vi "CVTTraceUpdate.vi"(8 "error in (no error)":errorcluster, 10 "Channels":string[](array[string]), 11 "TektronixDPOSimple in":refnum<class "Tektronix MDO MSO DPO.lvclass">) -> (0 "error out":errorcluster, 2 "CommandOut":string, 3 "TektronixDPOSimple out":refnum<class "Tektronix MDO MSO DPO.lvclass">)   [LabVIEW 2020, in "Tektronix MDO MSO DPO.lvclass"]
uses:
  Tektronix MDO MSO DPO.lvclass
  TraceGUI-Info.ctl
  Tektronix MDO MSO DPO.lvclass/Tektronix MDO MSO DPO.ctl
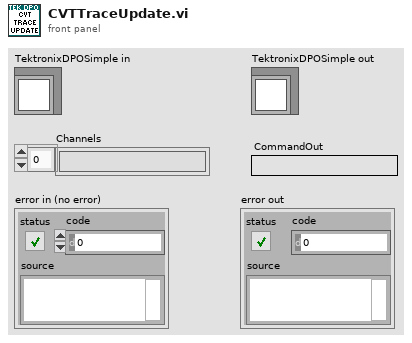
[diagram p1: front panel]
types:
  T1 = typedef "TraceGUI-Info.ctl" = cluster{"Number of channels":dbl, "GUInumPoints":i32}
  T2 = cluster{"Channel0":string, "Channel1":string, "Channel2":string, "Channel3":string, "Channel4":string, "Channel5":string, "Channel6":string, "Channel7":string}
  T3 = cluster{"actualSamples":i32, "absoluteInitialX":dbl, "relativeInitialX":dbl, "xIncrement":dbl, "offset":dbl, "gain":dbl, "reserved1":dbl, "reserved2":dbl}[]
  T4 = typedef "OnOffTypeDef.ctl" = enum16{"off", "on"}
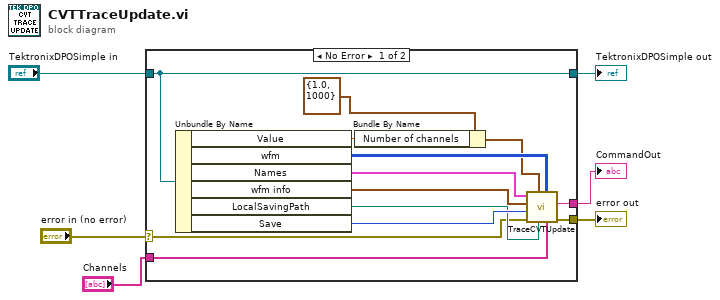
[diagram p0: block diagram]
diagram:
  n1 = case shown="No Error" "error in (no error)" {
    selector: "error in (no error)" -> [w11 w21]
    tunnel: [w14 w21] -> w6
    tunnel: [w13 _] -> w5
    tunnel: "Channels" -> [w12 _]
    tunnel: "TektronixDPOSimple in" -> [w10 w20]
    tunnel: [w10 w20] -> w1
    frame No Error {
      n2 = Unbundle By Name ("pressure read")(w10) -> ("Value"=w7:dbl, "wfm"=w19:i16[][], "Names"=w15:T2, "wfm info"=w18:T3, "LocalSavingPath"=w16:path, "Save"=w17:T4)
      n3 = Bundle By Name(cluster=T1 {"Number of channels"=1.0, "GUInumPoints"=1000} ("TraceGUI-Info"), "Number of channels"=w7) -> (w8:T1)
      n4 = call "TraceCVTUpdate.vi"("Channels"=w12, "wfm"=w19, "Settings.LocalSavingPath"=w16, "TraceGUI-Info"=w8, "error in (no error)"=w11, "Save"=w17, "wfm info"=w18, "Settings.Names"=w15) -> ("error out"=w14:errorcluster, "String out"=w13:string)  [unwired: 1 in, 1 out]
    }
    frame Error {
    }
  }
  "error out" <- w6
  "CommandOut" <- w5
  "TektronixDPOSimple out" <- w1
